vi "Drive Direction_Adam.vi"(7 "Wheels":T1=enum."Wheel 3", 8 "error in":errorcluster, 9 "Wheel Power":dbl format="%#_13g", 10 "Desired direction (radians)":dbl=6.283185307179586 format="%#_13g", 11 "Swerve":T1=enum."Swerve 3") -> (0 "error out":errorcluster)   [LabVIEW 2016]
uses:
  Refname/Motors.ctl
  Refname/Refname to String (Motors).vi
  Main/Robot Global Data.vi
  <vilib>/addons/control/pid/pid.llb/PID (DBL).vi
  <vilib>/addons/control/pid/NI_PID_pid.lvlib
panel:
  in  "PID gains":T2={"proportional gain (Kc)"=-0.0003125, "integral time (Ti, min)"=0.01, "derivative time (Td, min)"=0.0} {"derivative time (Td, min)" format="%.3f"; "integral time (Ti, min)" format="%.8f"; "proportional gain (Kc)" format="%.8f"}
  in  "output range":cluster{"output high":dbl, "output low":dbl}={"output high"=1.0, "output low"=-1.0}
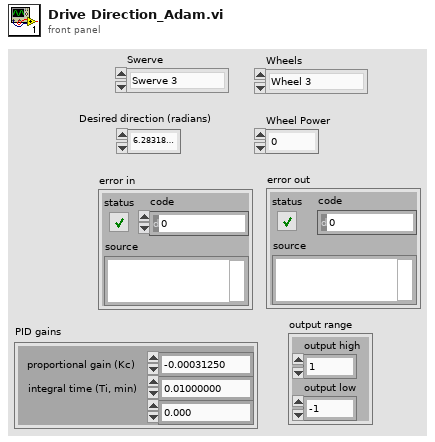
[diagram p1: front panel]
types:
  T1 = typedef "Motors.ctl" = enum16{"Wheel 1", "Swerve 1", "Wheel 2", "Swerve 2", "Wheel 3", "Swerve 3", "Wheel 4", "Swerve 4"}
  T2 = cluster{"proportional gain (Kc)":dbl, "integral time (Ti, min)":dbl, "derivative time (Td, min)":dbl}
  T3 = typedef "WPI_MotorControlDeviceRef.ctl" = cluster{"DeviceStatus":errorcluster, "Type":T4, "PWM":cluster{"PWM Channel":T5, "DeadBand":T6}, "CAN":cluster{"Device Number":u8, "SetOutput VI Ref":variant, "GetOutput VI Ref":variant, "Enable VI Ref":variant, "Disable VI Ref":variant, "Data":variant}, "Invert":bool}
  T4 = typedef "WPI_MotorControlType.ctl" = enum16{"PWM", "CAN"}
  T5 = typedef "FPGA_DIOPWMChannel.ctl" = enum8{"PWM 0", "PWM 1", "PWM 2", "PWM 3", "PWM 4", "PWM 5", "PWM 6", "PWM 7", "PWM 8", "PWM 9", "PWM MXP 0", "PWM MXP 1", "PWM MXP 2", "PWM MXP 3", "PWM MXP 4", "PWM MXP 5", "PWM MXP 6", "PWM MXP 7", "PWM MXP 8", "PWM MXP 9", "Invalid"}
  T6 = typedef "WPI_PWMDeadband.ctl" = cluster{"Name":string, "maxPositivePwm":i32, "minPositivePwm":i32, "centerPwm":i32, "maxNegativePwm":i32, "minNegativePwm":i32, "angularRange":u16}
  T7 = typedef "WPI_CANTalonSRX_GlobalStatus.ctl" = cluster{"Applied Throttle":dbl, "Module Enabled":bool, "CAN Error":errorcluster, "Closed Loop Error":dbl, "Forward Limit Switch Closed":bool, "Reverse Limit Switch Closed":bool, "Sensor Position":dbl, "Sensor Velocity":dbl, "Current":dbl, "Sticky Fault - Over Temp":bool, "Sticky Fault - Under Voltage":bool, "Sticky Fault - Forward Limit":bool, "Sticky Fault - Reverse Limit":bool, "Sticky Fault - Forward Soft Limit":bool, "Sticky Fault - Reverse Soft Limit":bool, "Brake is Enabled":bool, "Encoder Position":dbl, "Encoder Velocity":dbl, "Encoder Index Count":dbl, "Encoder A Pin State":bool, "Encoder B Pin State":bool, "Encoder Index Pin State":bool, "Analog In":dbl, "Analog In Velocity":dbl, "Temperature (C)":dbl, "Battery Voltage":dbl, "Control 5 Is Supported":bool, "Current Profile Slot Select":dbl, "Pos Div 8":bool, "Vel Div 4":bool, "Pulse Width Position":i32, "Pulse Width Velocity":i32, "Pulse Width Rise To Rise (us)":i32, "Pulse Width Rise To Fall (us)":i32, "Mot Prof Active Is Under Run":bool, "Mot Prof Active Has Under Run":bool, "Mot Prof Active Is Last":bool, "Mot Prof Active Velocity Only":bool, "Mot Prof Active Is Valid":bool, "Mot Prof Buffer Is Full":bool, "Mot Prof Active Profile Slot Select":i32, "Mot Prof NextID":i32, "Mot Prof Count":i32, "Mot Prof Active Velocity":dbl, "Mot Prof Active Position":dbl, "Mot Prof Output Enable":i32}
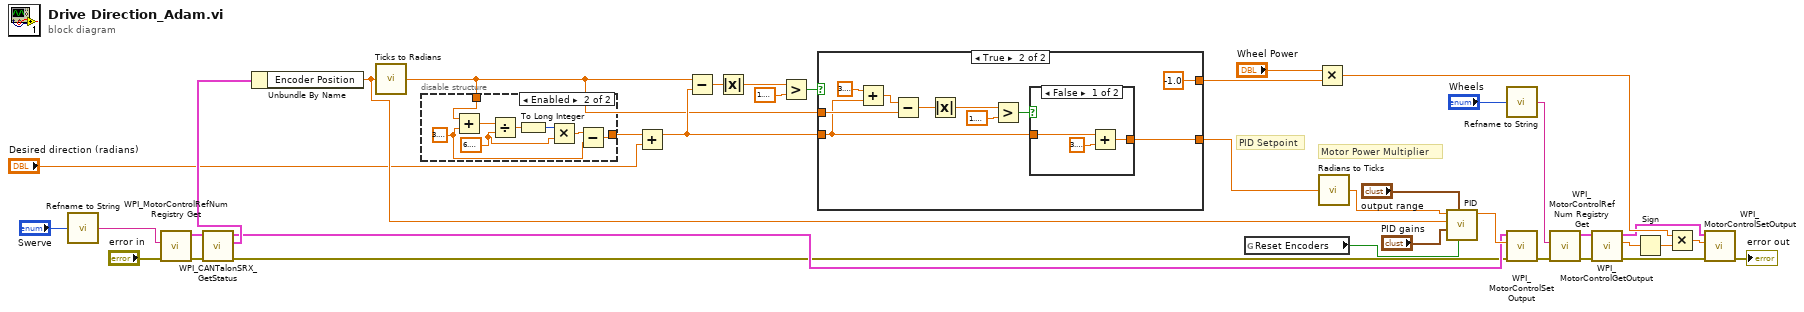
[diagram p0: block diagram]
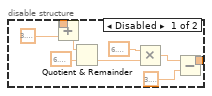
[diagram p2: hidden frame]
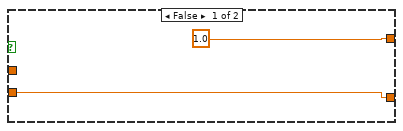
[diagram p3: hidden frame]
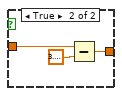
[diagram p4: hidden frame]
diagram:
  # "Motor Power Multiplier"
  # "PID Setpoint"
  n1 = call-poly "Refname to String.vi"("Enum"="Swerve") -> ("String"=w36:string)
  n2 = call <vilib>:"WPI_MotorControlRefNum Registry Get.vi"("error in (no error)"="error in", "refnum name"=w36) -> ("error out"=w33:errorcluster, "MotorControlDevRef"=w35:T3)  [unwired: 8 in]
  n3 = call <vilib>:"WPI_CANTalonSRX_GetStatus.vi"("error in (no error)"=w33, "CAN Talon SRX Ref"=w35) -> ("error out"=w4:errorcluster, "Talon SRX Status"=w31:T7, "CAN Talon SRX Ref"=w28:T3)  [unwired: 7 in]
  n4 = Unbundle By Name(w31) -> ("Encoder Position"=w14:dbl)
  n5 = call "Ticks to Radians.vi"("Ticks"=w14) -> ("Radians"=w2:dbl)
  n6 = disable-structure shown="Enabled" {
    disable-tunnel: w2 -> [w42 w54]
    disable-tunnel: [w39 w47] -> w1
    frame Disabled {
      n7 = Add(x=w42, y=3.141592653589793) -> (x+y=w41:dbl)
      n8 = Quotient & Remainder(x=w41, y=6.283185307179586) -> (floor(x/y)=w45:dbl)  [unwired: 1 out]
      n9 = Multiply(x=6.283185307179586, y=w45) -> (x*y=w43:dbl)
      n10 = Subtract(x=w43, y=3.141592653589793) -> (x-y=w39:dbl)
    }
    frame Enabled {
      w50 = 6.283185307179586
      w48 = 3.141592653589793
      n11 = Add(x=w54, y=w48) -> (x+y=w53:dbl)
      n12 = Divide(x=w53, y=w50) -> (x/y=w52:dbl)
      n13 = To Long Integer(number=w52) -> (32bit integer=w51:i32)
      n14 = Multiply(x=w51, y=w50) -> (x*y=w49:dbl)
      n15 = Subtract(x=w49, y=w48) -> (x-y=w47:dbl)
    }
  }
  n16 = Add(x=w1, y="Desired direction (radians)") -> (x+y=w13:dbl)
  n17 = Subtract(x=w2, y=w13) -> (x-y=w22:dbl)
  n18 = Absolute Value(x=w22) -> (abs(x)=w21:dbl)
  n19 = Greater?(x=w21, y=1.5707963267948966) -> (0:w20:bool)
  n20 = case shown="True" w20 {
    tunnel: [1.0 -1.0] -> w17
    tunnel: [w55 w58] -> w16
    tunnel: w13 -> [w55 w59]
    tunnel: w2 -> [_ w64]
    frame False {
    }
    frame True {
      n21 = Add(x=3.141592653589793, y=w59) -> (x+y=w65:dbl)
      n22 = Subtract(x=w65, y=w64) -> (x-y=w63:dbl)
      n23 = Absolute Value(x=w63) -> (abs(x)=w61:dbl)
      n24 = Greater?(x=w61, y=1.5707963267948966) -> (0:w66:bool)
      n25 = case shown="False" w66 {
        tunnel: w59 -> [w67 w71]
        tunnel: [w69 w70] -> w58
        frame False {
          n26 = Add(x=w67, y=3.141592653589793) -> (x+y=w69:dbl)
        }
        frame True {
          n27 = Subtract(x=w71, y=3.141592653589793) -> (x-y=w70:dbl)
        }
      }
    }
  }
  n28 = global read "Robot Global Data.vi" "Reset Encoders"() -> (w27:bool)
  n29 = Multiply(x="Wheel Power", y=w17) -> (x*y=w18:dbl)
  n30 = call "Radians to Ticks.vi"("Radians"=w16) -> ("Ticks"=w15:dbl)
  n31 = call-poly <vilib>:"PID.vi"("reinitialize? (F)"=w27, "output range"="output range", "PID gains"="PID gains", "process variable"=w14, "setpoint"=w15) -> ("output"=w29:dbl)  [unwired: 5 in, 1 out]
  n32 = call-poly "Refname to String.vi"("Enum"="Wheels") -> ("String"=w24:string)
  n33 = call <vilib>:"WPI_MotorControlSetOutput.vi"("error in (no error)"=w4, "Output"=w29, "MotorControlDevRef"=w28) -> ("error out"=w10:errorcluster)  [unwired: 6 in, 2 out]
  n34 = call <vilib>:"WPI_MotorControlRefNum Registry Get.vi"("error in (no error)"=w10, "refnum name"=w24) -> ("error out"=w6:errorcluster, "MotorControlDevRef"=w12:T3)  [unwired: 8 in]
  n35 = call <vilib>:"WPI_MotorControlGetOutput.vi"("error in"=w6, "MotorControlDevRef"=w12) -> ("error out"=w5:errorcluster, "Output"=w9:dbl, "MotorControlDevRef"=w11:T3)  [unwired: 7 in]
  n36 = Sign(1:w9) -> (0:w8:dbl)
  n37 = Multiply(x=w18, y=w8) -> (x*y=w7:dbl)
  n38 = call <vilib>:"WPI_MotorControlSetOutput.vi"("error in (no error)"=w5, "Output"=w7, "MotorControlDevRef"=w11) -> ("error out"=→"error out":errorcluster)  [unwired: 6 in, 2 out]
